vi "SVT UFF58 Read Record 7.vi"(0 "function refnum":refnum<k20>, 11 "error in (no error)":errorcluster) -> (4 "dup function refnum":refnum<k20>, 6 "data form":T1={"ordinate data type"=2, "number of data values/pairs"=0, "abscissa spacing"=enum."uneven", "abscissa minimum"=0.0, "abscissa increment"=0.0} {"ordinate data type" items=["real single precision"=2, "real double precision"=4, "complex single precision"=5, "complex double precision"=6]}, 15 "error out":errorcluster)   [LabVIEW 2017, in "SoundVib_UFF58.lvlib"]
doc: "Reads the values of all the fields in record 7 of a UFF58 (universal file format) file except field 6, z-axis value, which is not supported. Record 7 contains the data form."
uses:
  <vilib>/addons/Sound and Vibration/svt_UFF58/SoundVib_UFF58.lvlib
  <vilib>/addons/Sound and Vibration/svt_UFF58/subVIs/sv_UFF58 Data Form.ctl
  <vilib>/Platform/storage/Storage.llb/Get Property (DBL).vi
  <vilib>/Platform/storage/Storage.llb/Get Property (String).vi
  <vilib>/Platform/storage/Storage.llb/Get Property (Storage Refnums).vi
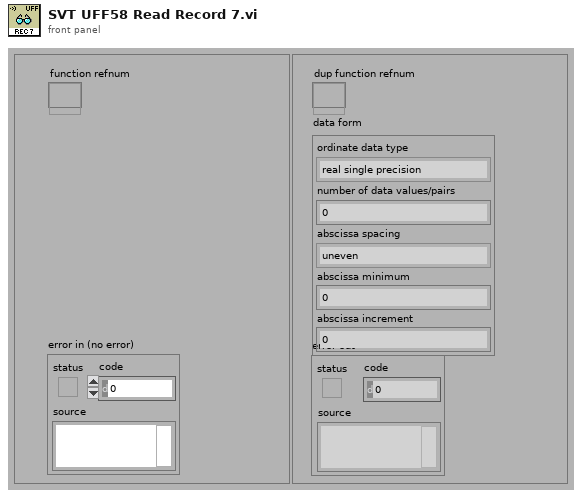
[diagram p1: front panel]
types:
  T1 = typedef "SoundVib_UFF58.lvlib/sv_UFF58 Data Form.ctl" = cluster{"ordinate data type":u16, "number of data values/pairs":i32, "abscissa spacing":enum16{"uneven", "even"}, "abscissa minimum":dbl, "abscissa increment":dbl}
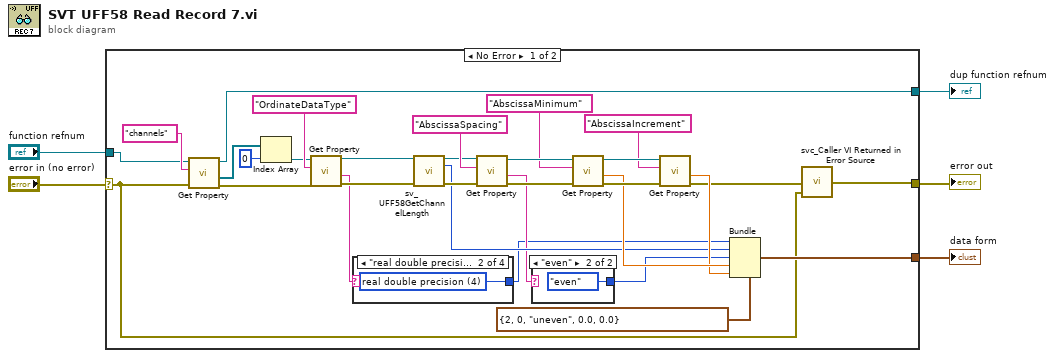
[diagram p0: block diagram]
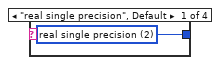
[diagram p2: hidden frame]
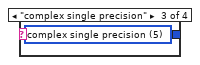
[diagram p3: hidden frame]
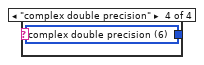
[diagram p4: hidden frame]
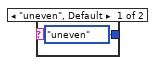
[diagram p5: hidden frame]
diagram:
  n1 = case shown="No Error" "error in (no error)" {
    selector: "error in (no error)" -> [w14 w43]
    tunnel: "function refnum" -> [w32 w44]
    tunnel: [w13 w44] -> w1
    tunnel: [w15 w43] -> w5
    tunnel: [w20 _] -> w4
    frame No Error {
      n2 = call-poly <vilib>:"Get Property.vi"("error in (no error)"=w14, "Property name"="channels", "storage refnum"=w32) -> ("error out"=w31:errorcluster, "Value"=w33:refnum<k20>[], "storage refnum out"=w13:refnum<k20>)  [unwired: 6 in]
      n3 = Index Array(array=w33, index=0) -> (element=w30:refnum<k20>)
      n4 = call-poly <vilib>:"Get Property.vi"("error in (no error)"=w31, "Property name"="OrdinateDataType", "storage refnum"=w30) -> ("error out"=w19:errorcluster, "Value"=w7:string, "storage refnum out"=w12:refnum<k20>)  [unwired: 6 in]
      n5 = case shown="\"real double precision\"" w7 {
        tunnel: [w37 w38 w39 w40] -> w6
        frame "real single precision", Default {
          w37 = u16 2 items=["real single precision"=2, "real double precision"=4, "complex single precision"=5, "complex double precision"=6] ("ordinate data type")
        }
        frame "real double precision" {
          w38 = u16 4 items=["real single precision"=2, "real double precision"=4, "complex single precision"=5, "complex double precision"=6] ("ordinate data type")
        }
        frame "complex single precision" {
          w39 = u16 5 items=["real single precision"=2, "real double precision"=4, "complex single precision"=5, "complex double precision"=6] ("ordinate data type")
        }
        frame "complex double precision" {
          w40 = u16 6 items=["real single precision"=2, "real double precision"=4, "complex single precision"=5, "complex double precision"=6] ("ordinate data type")
        }
      }
      n6 = call <vilib>:"sv_UFF58GetChannelLength.vi"("channel refnum"=w12, "error in"=w19) -> ("dup channel refnum"=w18:refnum<k20>, "channel length"=w16:i32, "error out"=w17:errorcluster)  [unwired: 11 in]
      n7 = call-poly <vilib>:"Get Property.vi"("error in (no error)"=w17, "Property name"="AbscissaSpacing", "storage refnum"=w18) -> ("error out"=w27:errorcluster, "Value"=w9:string, "storage refnum out"=w28:refnum<k20>)  [unwired: 6 in]
      n8 = case shown="\"even\"" w9 {
        tunnel: [enum16{"uneven", "even"}."uneven" ("abscissa spacing") enum16{"uneven", "even"}."even" ("abscissa spacing")] -> w8
        frame "uneven", Default {
        }
        frame "even" {
        }
      }
      n9 = call-poly <vilib>:"Get Property.vi"("error in (no error)"=w27, "Property name"="AbscissaMinimum", "storage refnum"=w28) -> ("error out"=w25:errorcluster, "Value"=w22:dbl, "storage refnum out"=w26:refnum<k20>)  [unwired: 6 in]
      n10 = call-poly <vilib>:"Get Property.vi"("error in (no error)"=w25, "Property name"="AbscissaIncrement", "storage refnum"=w26) -> ("error out"=w11:errorcluster, "Value"=w21:dbl)  [unwired: 6 in, 1 out]
      n11 = Bundle(cluster=T1 {"ordinate data type"=2, "number of data values/pairs"=0, "abscissa spacing"=enum."uneven", "abscissa minimum"=0.0, "abscissa increment"=0.0} ("data form"), "ordinate data type"=w6, "number of data values/pairs"=w16, "abscissa spacing"=w8, "abscissa minimum"=w22, "abscissa increment"=w21) -> (w20:T1)
      n12 = call <vilib>:"svc_Caller VI Returned in Error Source.vi"("warning input to caller"=w14, "error in (no error)"=w11) -> ("error out"=w15:errorcluster)  [unwired: 3 in]
    }
    frame Error {
    }
  }
  "error out" <- w5
  "data form" <- w4
  "dup function refnum" <- w1
